vi "Moving_average.vi"(10 "average length":i32=100, 11 "Input":dbl[](array[numeric])) -> (3 "Output":dbl[](array[numeric]))   [LabVIEW 2020]
uses:
  <vilib>/Analysis/baseanly.llb/Mean (DBL).vi
  <vilib>/Analysis/NI_AALBase.lvlib
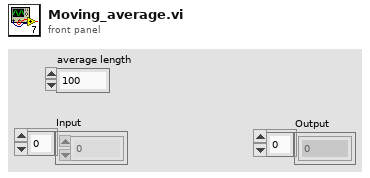
[diagram p1: front panel]
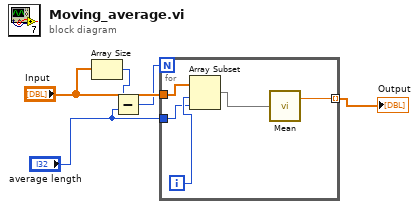
[diagram p0: block diagram]
diagram:
  n1 = Array Size(array="Input") -> (size(s)=w4:i32)
  n2 = Subtract(x=w4, y="average length") -> (x-y=w2:i32)
  n3 = for {
    N: w2 -> [_]
    tunnel: "average length" -> [w8]
    tunnel: "Input" -> [w10]
    tunnel: [w6] -> w1 mode=indexing
    i -> [w9]
    n4 = Array Subset(array=w10, index=w9, length=w8) -> (w7:dbl[])
    n5 = call-poly <vilib>:"Mean.vi"("X"=w7) -> ("mean"=w6:dbl)  [unwired: 1 out]
  }
  "Output" <- w1
